vi "Diagnostics.Main.UUDT.Engine.vi"(8 "error in (no error)":errorcluster, 11 "State Variables":T1={"Comm"=refnum, "Parameters"={"Properties"={"Name"="", "CAN"={"CAN Interface"=enum."CAN1", "Baud Rate"=0, "Diagnostic Protocol"=enum."GMLAN", "Transport Protocol"=enum."ISO TP - Normal Mode", "Transmit ID"=0, "Receive ID"=0, "Transmit Extension"=2, "Receive Extension"=1, "Receive UUDT ID"=0, "Enable Stream"=TRUE, "VW TP Channel ID"=0, "Security"={"Source DLL Path"=path "", "Security Level"=0, "Target DLL Path"=path ""}, "Fill Frame"=FALSE, "Fill Byte"=255, "Termination"=FALSE}, "986x"={"Enable"=FALSE, "RIO Device"=0, "Bitfile"=path ""}, "Reads"=[], "Frames Lookup"=variant(enum16{"GMLAN", "KWP-2000", "UDS"} enum."GMLAN"), "Writes"=[], "DPIDs"=[], "DPID Lookup"=variant(u32 0), "DTC descriptor"={"DTC Byte Length"=2, "Status Byte Length"=1, "Add Data Byte Length"=1, "Byte Order"=enum."Motorola"}, "Created DTCs"=0}}, "ADCS Connection"={"Diag CAN Handle"=0, "Transport Protocol"=enum."ISO TP - Normal Mode", "Receive Address Extension"=0, "Transmit Address Extension"=0, "Receive CAN Id"=0, "Transmit CAN Id"=0, "Diag CAN Queue"=refnum, "Log Frames ?"=FALSE, "My TP Address"=0, "Other TP Address"=0, "T1"=0, "T2"=0, "T3"=0, "T4"=0, "Tx SN"=0, "Block Size"=0, "Rx SN"=0, "VW TP Initialized?"=FALSE, "Tx block no"=0, "baud rate"=0, "Interface"="", "Channel Diag CAN Handle"=0, "UDP Connection ID"=refnum, "TCP Connection ID"=refnum, "Target IP Addr"=0, "Source Address"=0, "Target Address"=0, "Send Header NACK?"=FALSE, "DLL Handle"=0, "NAD"=0, "Time Stamp read first"=0.0, "Time Stamp read last"=0.0, "Time Stamp write first"=0.0, "Time Stamp write last"=0.0, "Time Stamp write"=0.0, "Time Stamp read"=0.0}, "XNET References"={"Database"="", "GMLAN DPID Session"="", "Cluster"=""}, "XNETEngine (GMLAN)"=refnum, "Process"=refnum, "Reads"=refnum, "Writes"=refnum, "Cmds"=refnum, "DTCs"=refnum, "DTC Count"=refnum, "Status"=refnum, "Triggers"=refnum} {"Parameters"."Properties"."Writes"."Signals"."Byte Order" items=["Little Endian", "Big Endian"]; "Parameters"."Properties"."Writes"."Signals"."Data Type" items=["Signed", "Unsigned", "IEEE Float"]; "Parameters"."Properties"."CAN"."Fill Byte" format="%.0x"; "Parameters"."Properties"."CAN"."VW TP Channel ID" format="%.0x"; "Parameters"."Properties"."CAN"."Receive UUDT ID" format="%.0x"; "Parameters"."Properties"."CAN"."Receive Extension" format="%.0x"; "Parameters"."Properties"."CAN"."Transmit Extension" format="%.0x"; "Parameters"."Properties"."CAN"."Receive ID" format="%.0x"; "Parameters"."Properties"."CAN"."Transmit ID" format="%.0x"; "Parameters"."Properties"."Reads"."Signals"."Byte Order" items=["Little Endian", "Big Endian"]; "Parameters"."Properties"."Reads"."Signals"."Data Type" items=["Signed", "Unsigned", "IEEE Float"]}) -> (0 "error out":errorcluster)   [LabVIEW 2015, in "Diagnostics Addon Engine.lvlib"]
uses:
  Diagnostics Addon Engine.lvlib
  Types/Diagnostics.State.ctl
  <vilib>/NI/NIVS Inline Async API/_VS Inline Async API/Process/Process.lvclass
  <vilib>/NI/NIVS Addon Network Comm/Engine/VeriStand Comm.lvclass
  Shared/Types/SysDef.Compile.ctl
  Shared/Types/SysDef.Compile.Properties.ctl
  Shared/Types/CAN.ctl
  Shared/Types/CAN.Interface.ctl
  Shared/Types/Protocol.ctl
  Shared/Types/Transport.ctl
  Shared/Types/Security.ctl
  Shared/Types/986x.ctl
  Shared/Types/Frame.Compile.ctl
  Shared/Types/Type.ctl
  Shared/Types/Signal.ctl
  Shared/Types/DPID.ctl
  Shared/Types/DPID.Rate.ctl
  Shared/Types/DTCDescriptor.ctl
  <vilib>/Automotive Diagnostic Command Set/Diagnostic Transport.llb/Diag Reference.ctl
  <vilib>/Automotive Diagnostic Command Set/Diagnostic Transport.llb/Transport Protocol Selector.ctl
  <vilib>/Automotive Diagnostic Command Set/Diagnostic Transport.llb/Diag CAN Frame Log.ctl
  Types/XNET.Refs.ctl
  <vilib>/NI/AMC/Message Queue.ctl
  <vilib>/NI/AMC/Message.ctl
  <vilib>/NI/Tools/Keyed Array/KeyedArray.ctl
  <vilib>/NI/NIVS Inline Async API/_Data Access Engine/Data Access Engine/Types/Write.DVR.ctl
  <vilib>/NI/NIVS Inline Async API/_Data Access Engine/Access Type Classes/Write/Write.lvclass
  <vilib>/NI/NIVS Inline Async API/_Data Access Engine/Data Access Engine/Types/Read.DVR.ctl
  <vilib>/NI/NIVS Inline Async API/_Data Access Engine/Access Type Classes/Read/Read.lvclass
  <vilib>/NI/NIVS Inline Async API/_Data Access Engine/Data Access Engine/Types/ReadWrite.DVR.ctl
  <vilib>/NI/NIVS Inline Async API/_Data Access Engine/Access Type Classes/ReadWrite/ReadWrite.lvclass
  Types/DTC.ChangeCount.Info.ctl
  Shared/Types/DTC.Info.ctl
  <vilib>/xnet/xnet.llb/XNET Frame CAN.ctl
  <vilib>/xnet/xnet.llb/XNET Frame Type CAN.ctl
  <vilib>/NI/NIVS Inline Async API/_Data Access Engine/Access Type Classes/Write/Write.lvclass/Write.ctl
  Types/Frame.Data.ctl
  Shared/Types/DPID.Lookup.Info.ctl
  Shared/Types/DPID.Lookup.Info.PID.ctl
  Shared/Types/Frame.Lookup.Info.ctl
  <vilib>/NI/NIVS Addon Network Comm/Engine/VeriStand Comm.lvclass/VeriStand Comm.ctl
  <vilib>/NI/NIVS Inline Async API/_VS Inline Async API/Process/Process.lvclass/Process.ctl
  <vilib>/NI/NIVS Inline Async API/_Data Access Engine/Data Access Engine/Methods/Write.Data.vi
  <vilib>/NI/NIVS Inline Async API/_Data Access Engine/Data Access Engine/Methods/Write.Data.Commit.vi
  <vilib>/NI/NIVS Inline Async API/_Data Access Engine/Data Access Engine/Methods/Write.Data.Buffer.vi
  <vilib>/NI/NIVS Inline Async API/_Data Access Engine/Access Type Classes/Write/Write.ProcessData.vi
  <vilib>/NI/NIVS Inline Async API/_Data Access Engine/Access Type Classes/Write/Write.Commit.vi
  <vilib>/NI/NIVS Inline Async API/_Data Access Engine/Access Type Classes/Write/Write.Buffer.vi
  GMLAN/Utilities/Convert Raw Data to DTCs.vi
  <vilib>/NI/AMC/Send Local Message.vi
  <vilib>/NI/AMC/Read Termination Message.vi
  <vilib>/NI/NIVS Inline Async API/_VS Inline Async API/Error Handling Process/SubVIs/Error.ConvertArray.vi
  <vilib>/NI/AMC/Create Single Message.vi
  <vilib>/NI/AMC/Update Message Routing Info.vi
  <vilib>/NI/AMC/Send Message.vi
  <vilib>/Automotive Diagnostic Command Set/Diagnostic Protocols.llb/Convert to Phys.vi
  <vilib>/xnet/xnet.llb/XNET Convert (Frame Raw to Signal).vi
  <vilib>/xnet/xnet.llb/XNET Read (Frame CAN).vi
  <vilib>/xnet/xnet.llb/XNET Convert (Frame CAN to Signal).vi
  Shared/SubVIs/Constants.vi
  <vilib>/NI/AMC/Globals.vi
  Shared/Diagnostics Addon Shared.lvlib
  <vilib>/NI Veristand/Custom Device Tools/Custom Device Utility Library/Custom Device Utility Library.lvlib
  <vilib>/NI/AMC/AMC.lvlib
  GMLAN/GMLAN.lvlib
  <vilib>/NI/NIVS Inline Async API/_Data Access Engine/Data Access Engine/Data Access Engine.lvclass
  <vilib>/NI/Tools/Keyed Array/Tools_KeyedArray.lvlib
  <vilib>/addons/Automotive Diagnostic Command Set/NI_Automotive Diagnostic Command Set.lvlib
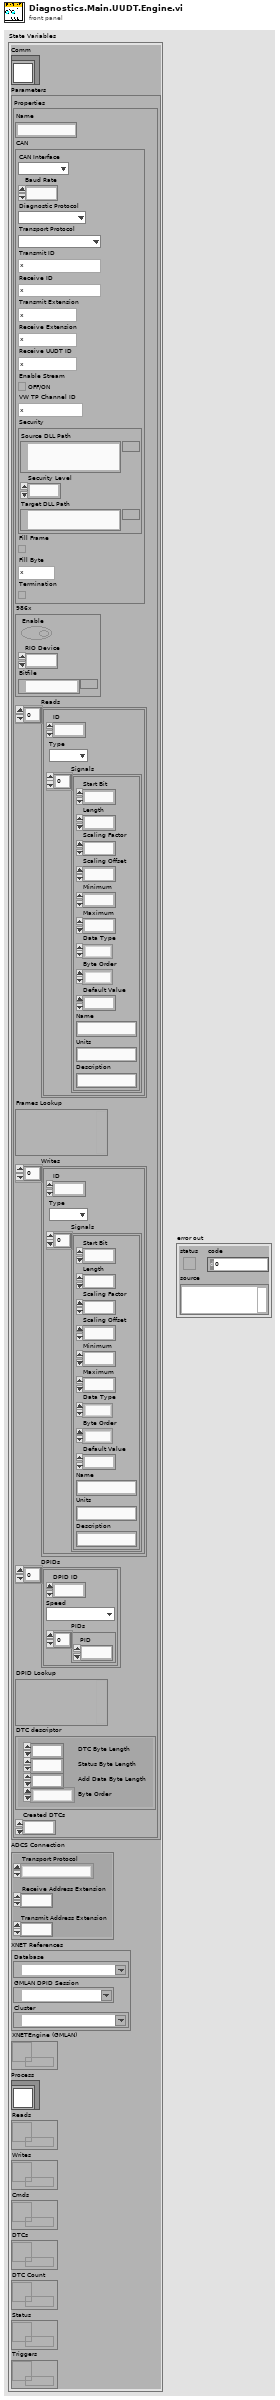
[diagram p1: front panel]
types:
  T1 = typedef "Diagnostics Addon Engine.lvlib/Diagnostics.State.ctl" = cluster{"Comm":refnum<class "VeriStand Comm.lvclass">, "Parameters":T2, "ADCS Connection":T16, "XNET References":T18, "XNETEngine (GMLAN)":T19, "Process":refnum<class "Process.lvclass">, "Reads":T20, "Writes":T21, "Cmds":T22, "DTCs":T20, "DTC Count":T20, "Status":T20, "Triggers":T22}
  T2 = typedef "Diagnostics Addon Shared.lvlib/SysDef.Compile.ctl" = cluster{"Properties":T3}
  T3 = typedef "Diagnostics Addon Shared.lvlib/SysDef.Compile.Properties.ctl" = cluster{"Name":string, "CAN":T4, "986x":T9, "Reads":T10[], "Frames Lookup":variant, "Writes":T10[], "DPIDs":T13[], "DPID Lookup":variant, "DTC descriptor":T15, "Created DTCs":u32}
  T4 = typedef "Diagnostics Addon Shared.lvlib/CAN.ctl" = cluster{"CAN Interface":T5, "Baud Rate":u32, "Diagnostic Protocol":T6, "Transport Protocol":T7, "Transmit ID":u32, "Receive ID":u32, "Transmit Extension":u8, "Receive Extension":u8, "Receive UUDT ID":u32, "Enable Stream":bool, "VW TP Channel ID":u32, "Security":T8, "Fill Frame":bool, "Fill Byte":u8, "Termination":bool}
  T5 = typedef "Diagnostics Addon Shared.lvlib/CAN.Interface.ctl" = enum16{"CAN0", "CAN1", "CAN2", "CAN3", "CAN4", "CAN5", "CAN6", "CAN7", "CAN8", "CAN9", "CAN10", "CAN11", "CAN12", "CAN13", "CAN14", "CAN15", "CAN16", "CAN17", "CAN18", "CAN19", "CAN20", "CAN21", "CAN22", "CAN23", "CAN24", "CAN25", "CAN26", "CAN27", "CAN28", "CAN29", "CAN30", "CAN31", "CAN32", "CAN33", "CAN34", "CAN35", "CAN36", "CAN37", "CAN38", "CAN39", "CAN40", "CAN41", "CAN42", "CAN43", "CAN44", "CAN45", "CAN46", "CAN47", "CAN48", "CAN49", "CAN50", "CAN51", "CAN52", "CAN53", "CAN54", "CAN55", "CAN56", "CAN57", "CAN58", "CAN59", "CAN60", "CAN61", "CAN62", "CAN63", "CAN 256 (Virtual)", "CAN 257 (Virtual)"}
  T6 = typedef "Diagnostics Addon Shared.lvlib/Protocol.ctl" = enum16{"GMLAN", "KWP-2000", "UDS", "User-Defined"}
  T7 = typedef "Diagnostics Addon Shared.lvlib/Transport.ctl" = enum16{"ISO TP - Normal Mode", "ISO TP - Mixed Mode", "VW TP 2.0", "Diagnostics on IP"}
  T8 = typedef "Diagnostics Addon Shared.lvlib/Security.ctl" = cluster{"Source DLL Path":path, "Security Level":u8, "Target DLL Path":path}
  T9 = typedef "Diagnostics Addon Shared.lvlib/986x.ctl" = cluster{"Enable":bool, "RIO Device":u16, "Bitfile":path}
  T10 = typedef "Diagnostics Addon Shared.lvlib/Frame.Compile.ctl" = cluster{"ID":u32, "Type":T11, "Signals":T12[]}
  T11 = typedef "Diagnostics Addon Shared.lvlib/Type.ctl" = enum16{"DID", "CDID", "PID", "CPID", "Read Memory", "Write Memory", "DTC Control", "IO Cmd", "IO Resp", "Routine Start Cmd", "Routine Start Resp", "Routine Request Cmd", "Routine Request Resp", "Routine Stop Cmd", "Routine Stop Resp", "UserDefined Cmd", "UserDefined Rsp"}
  T12 = typedef "Diagnostics Addon Shared.lvlib/Signal.ctl" = cluster{"Start Bit":u32, "Length":u32, "Scaling Factor":dbl, "Scaling Offset":dbl, "Minimum":dbl, "Maximum":dbl, "Data Type":u32, "Byte Order":u32, "Default Value":dbl, "Name":string, "Units":string, "Description":string}
  T13 = typedef "Diagnostics Addon Shared.lvlib/DPID.ctl" = cluster{"DPID ID":u8, "Speed":T14, "PIDs":u16[]}
  T14 = typedef "Diagnostics Addon Shared.lvlib/DPID.Rate.ctl" = enum16{"Slow", "Medium", "Fast"}
  T15 = typedef "Diagnostics Addon Shared.lvlib/DTCDescriptor.ctl" = cluster{"DTC Byte Length":i32, "Status Byte Length":i32, "Add Data Byte Length":i32, "Byte Order":enum16{"Motorola", "Intel"}}
  T16 = typedef "NI_Automotive Diagnostic Command Set.lvlib/Diag Reference.ctl" = cluster{"Diag CAN Handle":u32, "Transport Protocol":T17, "Receive Address Extension":u8, "Transmit Address Extension":u8, "Receive CAN Id":u32, "Transmit CAN Id":u32, "Diag CAN Queue":refnum<queue>, "Log Frames ?":bool, "My TP Address":u8, "Other TP Address":u8, "T1":u16, "T2":u16, "T3":u16, "T4":u16, "Tx SN":u8, "Block Size":u8, "Rx SN":u8, "VW TP Initialized?":bool, "Tx block no":u8, "baud rate":u32, "Interface":string, "Channel Diag CAN Handle":u32, "UDP Connection ID":refnum<k16>, "TCP Connection ID":refnum<k5>, "Target IP Addr":u32, "Source Address":u16, "Target Address":u16, "Send Header NACK?":bool, "DLL Handle":u32, "NAD":u8, "Time Stamp read first":dbl, "Time Stamp read last":dbl, "Time Stamp write first":dbl, "Time Stamp write last":dbl, "Time Stamp write":dbl, "Time Stamp read":dbl}
  T17 = typedef "NI_Automotive Diagnostic Command Set.lvlib/Transport Protocol Selector.ctl" = enum16{"ISO TP - Normal Mode", "ISO TP - Mixed Mode", "VW TP 2.0", "Diagnostics on IP", "ISO TP LIN"}
  T18 = typedef "Diagnostics Addon Engine.lvlib/XNET.Refs.ctl" = cluster{"Database":refnum<k21>, "GMLAN DPID Session":refnum<k21>, "Cluster":refnum<k21>}
  T19 = typedef "AMC.lvlib/Message Queue.ctl" = refnum<queue>
  T20 = typedef "Data Access Engine.lvlib/Data Access Engine.lvclass/Write.DVR.ctl" = refnum<data-value>
  T21 = typedef "Data Access Engine.lvlib/Data Access Engine.lvclass/Read.DVR.ctl" = refnum<data-value>
  T22 = typedef "Data Access Engine.lvlib/Data Access Engine.lvclass/ReadWrite.DVR.ctl" = refnum<data-value>
  T23 = typedef "Diagnostics Addon Shared.lvlib/DTC.Info.ctl" = cluster{"Timestamp":dbl, "DTC":dbl, "Status":dbl, "Add Data":dbl}
  T24 = typedef "Diagnostics Addon Engine.lvlib/DTC.ChangeCount.Info.ctl" = cluster{"DTCCountChange?":bool, "Timestamp":timestamp}
  T25 = typedef "XNET Frame CAN.ctl" = cluster{"timestamp":timestamp, "payload":u8[], "identifier":u32, "type":T26, "extended?":bool, "echo?":bool}
  T26 = typedef "XNET Frame Type CAN.ctl" = u8
  T27 = cluster{"Change DTC Count Cluster":T24, "Previous DTCs":T23[], "Prev DTC Frames":T25[]}
  T28 = typedef "Diagnostics Addon Engine.lvlib/Frame.Data.ctl" = cluster{"ID":u16, "Raw Frame":u8[]}
  T29 = typedef "Diagnostics Addon Shared.lvlib/DPID.Lookup.Info.ctl" = cluster{"PID Info":T30, "Datatable Lookup":T31, "Conversion":refnum<k21>}
  T30 = typedef "Diagnostics Addon Shared.lvlib/DPID.Lookup.Info.PID.ctl" = cluster{"PID":u16, "Frame Length":u8}
  T31 = typedef "Diagnostics Addon Shared.lvlib/Frame.Lookup.Info.ctl" = cluster{"Offset":i32, "Length":i32, "ByteLength":u16}
  T32 = typedef "Diagnostic Trouble Code.ctl" = cluster{"DTC":u32, "Status":u32, "Add Data":u32}
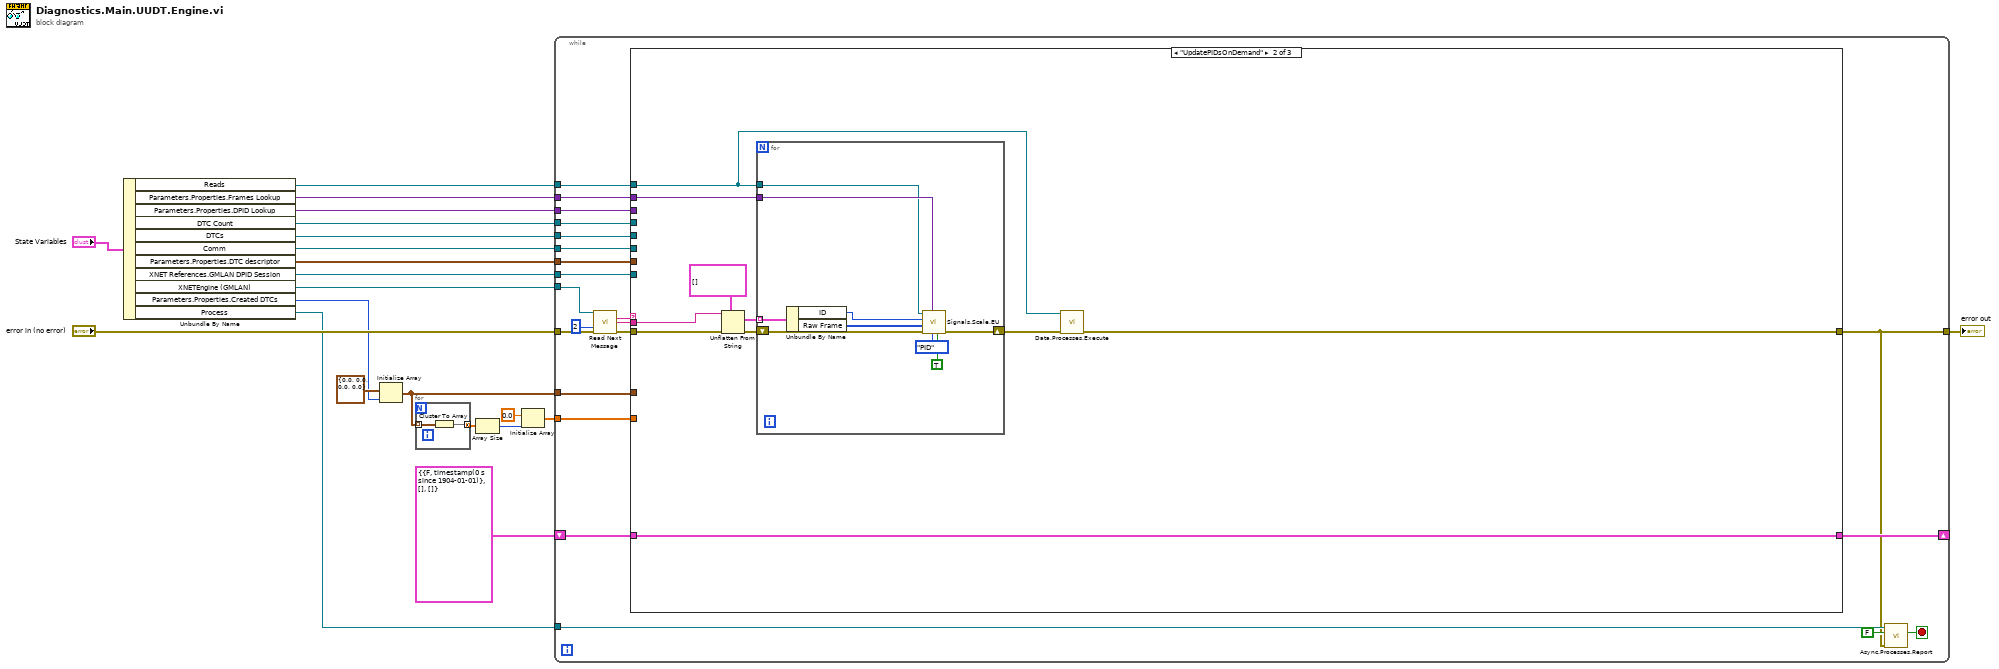
[diagram p0: block diagram]
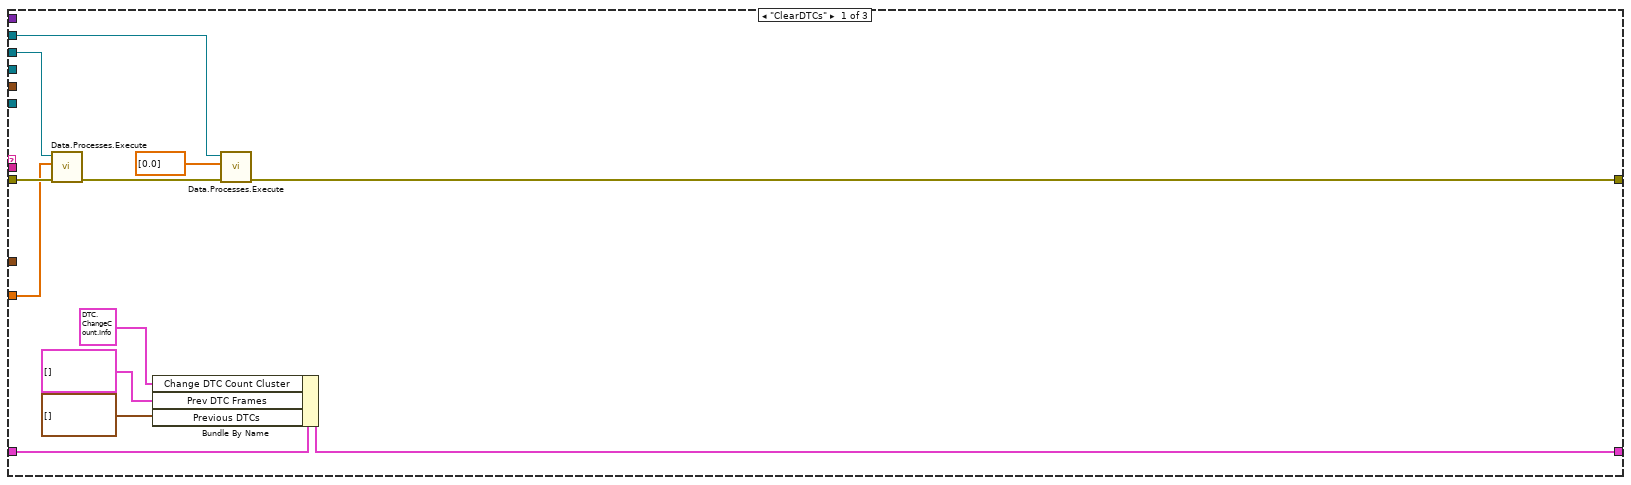
[diagram p2: hidden frame]
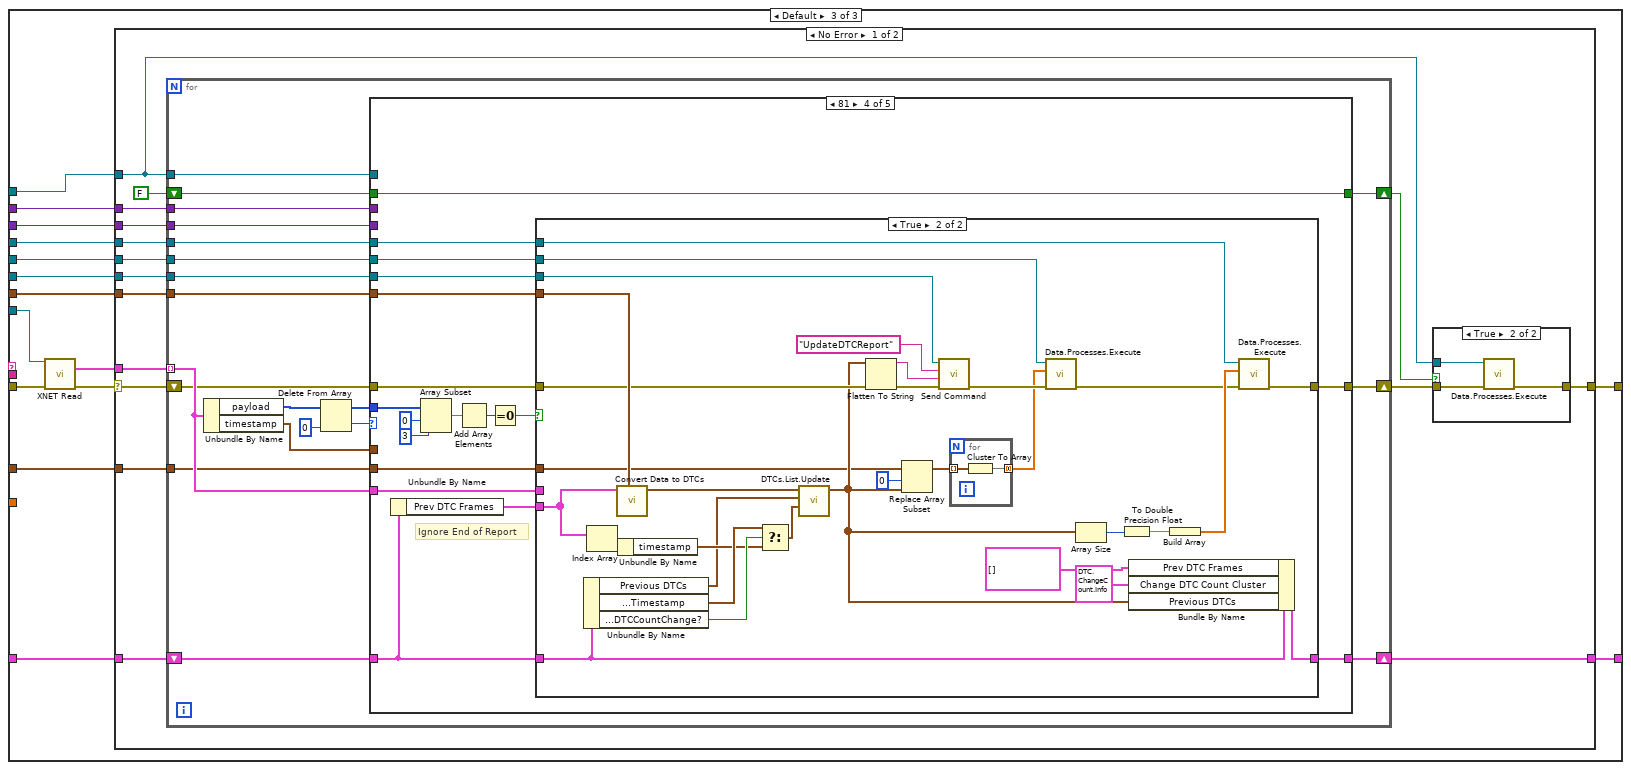
[diagram p3: hidden frame]
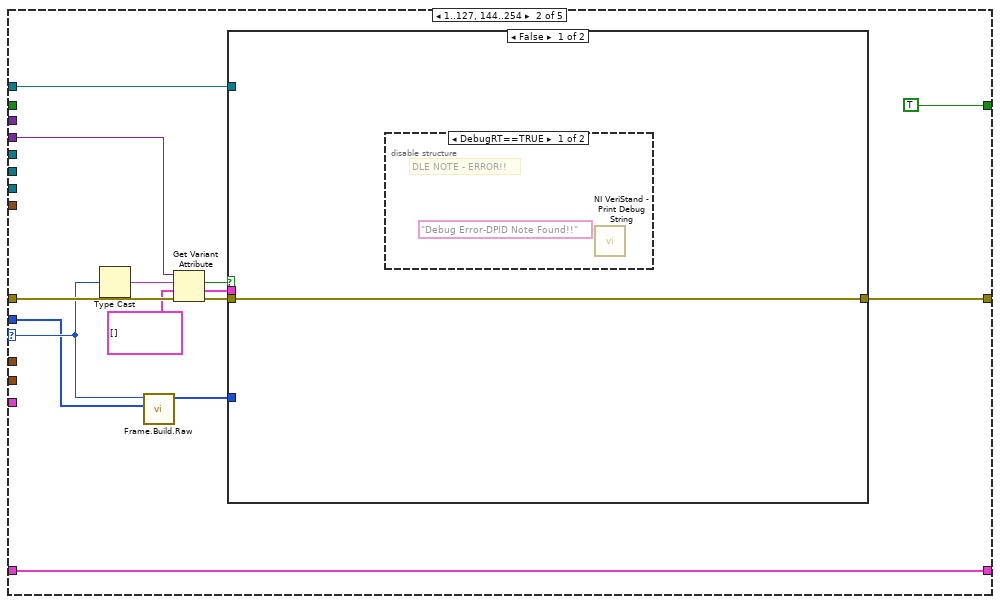
[diagram p5: hidden frame]
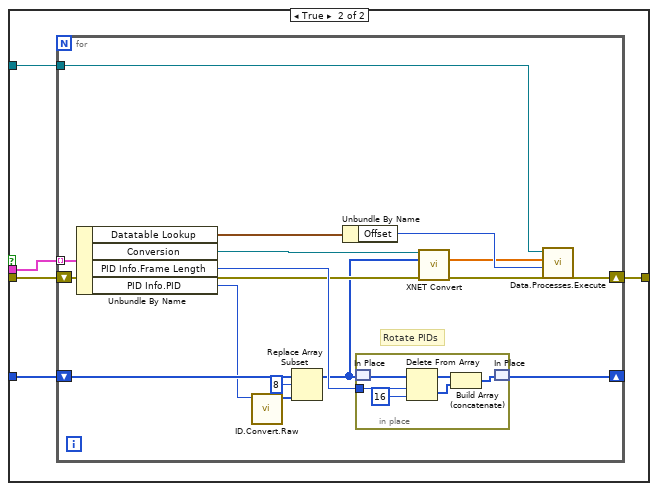
[diagram p7: hidden frame]
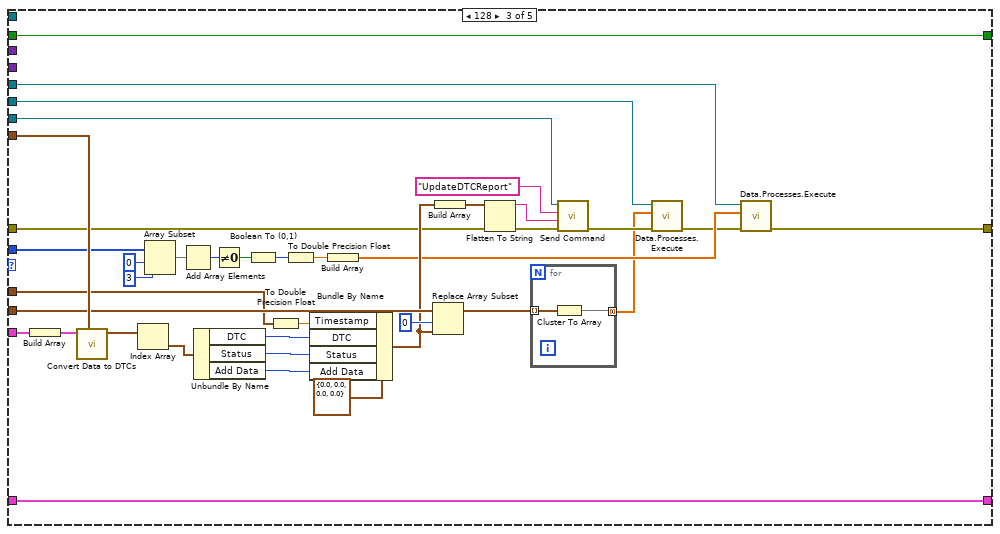
[diagram p8: hidden frame]
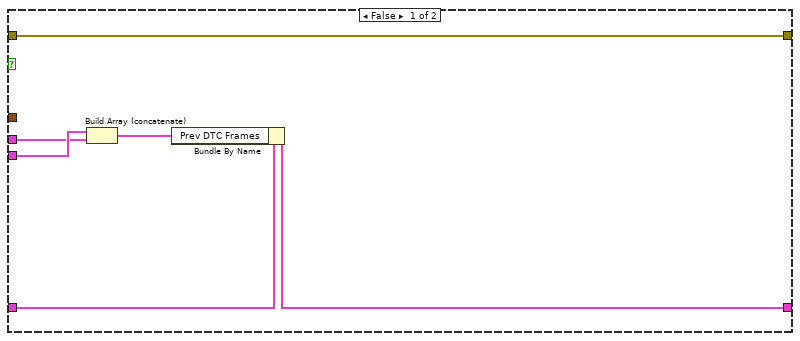
[diagram p9: hidden frame]
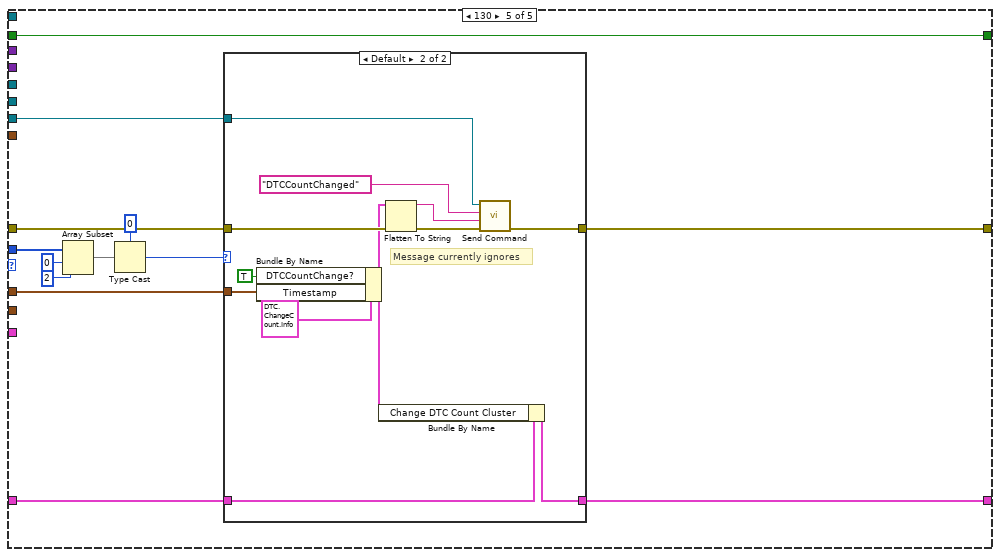
[diagram p10: hidden frame]
diagram:
  n1 = Unbundle By Name("State Variables") -> ("Reads"=w16:T20, "Parameters.Properties.Frames Lookup"=w15:variant, "Parameters.Properties.DPID Lookup"=w9:variant, "DTC Count"=w11:T20, "DTCs"=w19:T20, "Comm"=w18:refnum<class "VeriStand Comm.lvclass">, "Parameters.Properties.DTC descriptor"=w12:T15, "XNET References.GMLAN DPID Session"=w14:refnum<k21>, "XNETEngine (GMLAN)"=w8:T19, "Parameters.Properties.Created DTCs"=w7:u32, "Process"=w1:refnum<class "Process.lvclass">)
  n2 = Initialize Array(T23 {"Timestamp"=0.0, "DTC"=0.0, "Status"=0.0, "Add Data"=0.0} ("Diagnostic Trouble Code"), w7) -> (w6:T23[])
  n3 = for {
    tunnel: w6 -> [w23] mode=indexing
    tunnel: [w22] -> w3 mode=concatenating
    n4 = Cluster To Array(cluster=w23) -> (array=w22:dbl[])
  }
  n5 = Array Size(array=w3) -> (size(s)=w4:i32)
  n6 = Initialize Array(0.0 ("element"), w4) -> (w2:dbl[])
  n7 = while {
    tunnel: "error in (no error)" -> [w39]
    tunnel: [w26] -> w13
    tunnel: w12 -> [w45]
    tunnel: w14 -> [w44]
    tunnel: w15 -> [w43]
    tunnel: w16 -> [w42]
    tunnel: w18 -> [w41]
    tunnel: w1 -> [w28]
    tunnel: w8 -> [w33]
    shift-right: [w35] -> _
    shift-left: T27 {"Change DTC Count Cluster"={"DTCCountChange?"=FALSE, "Timestamp"=timestamp(0 s since 1904-01-01)}, "Previous DTCs"=[], "Prev DTC Frames"=[]} -> [w36]
    tunnel: w19 -> [w34]
    tunnel: w11 -> [w32]
    tunnel: w6 -> [w31]
    tunnel: w9 -> [w30]
    tunnel: w2 -> [w24]
    stop <- w25 stop-if-true
    n8 = call <vilib>:"Read Next Message.vi"("message queue in"=w33, "timeout (1 ms)"=2 ("timeout (1ms)"), "error in"=w39) -> ("message name"=w37:string, "message value"=w29:string, "error out"=w38:errorcluster)  [unwired: 5 in, 5 out]
    n9 = case shown="\"UpdatePIDsOnDemand\"" w37 {
      tunnel: [w48 w59 w89] -> w26
      tunnel: w45 -> [_ _ w88]
      tunnel: w38 -> [w47 w67 w87]
      tunnel: w44 -> [_ _ w86]
      tunnel: w43 -> [_ w62 w85]
      tunnel: w42 -> [_ w58 w84]
      tunnel: w41 -> [_ _ w83]
      tunnel: w36 -> [w57 w61 w82]
      tunnel: [w56 w61 w81] -> w35
      tunnel: w34 -> [w52 _ w80]
      tunnel: w32 -> [w50 _ w79]
      tunnel: w31 -> [_ _ w78]
      tunnel: w30 -> [_ _ w77]
      tunnel: w29 -> [_ w66 _]
      tunnel: w24 -> [w46 _ _]
      frame "ClearDTCs" {
        n10 = call-poly <vilib>:"Data.Processes.Execute.vi"("error in (no error)"=w47, "Values"=w46, "Ref"=w52) -> ("error out"=w49:errorcluster)  [unwired: 8 in]
        n11 = Bundle By Name(cluster=w57, "Change DTC Count Cluster"=T24 {"DTCCountChange?"=FALSE, "Timestamp"=timestamp(0 s since 1904-01-01)}, "Prev DTC Frames"=T25[] [] ("Previous DTC Frames"), "Previous DTCs"=T23[] []) -> (w56:T27)
        n12 = call-poly <vilib>:"Data.Processes.Execute.vi"("error in (no error)"=w49, "Values"=dbl[] [0.0] ("element"), "Ref"=w50) -> ("error out"=w48:errorcluster)  [unwired: 8 in]
      }
      frame "UpdatePIDsOnDemand" {
        n13 = Unflatten From String(type=T28[] [], binary string=w66, error in (no error)=w67) -> (value=w63:T28[], error out=w64:errorcluster)  [unwired: 2 in, 1 out]
        n14 = for {
          shift-right: [w72] -> w60
          shift-left: w64 -> [w73]
          tunnel: w63 -> [w76] mode=indexing
          tunnel: w62 -> [w71]
          tunnel: w58 -> [w69]
          n15 = Unbundle By Name(w76) -> ("ID"=w75:u16, "Raw Frame"=w74:u8[])
          n16 = call "Signals.Scale.EU.vi"("Buffer?"=TRUE, "Type"=Type."PID", "Lookup"=w71, "error in (no error)"=w73, "Unscaled Data"=w74, "ID"=w75, "Reads Ref"=w69) -> ("error out"=w72:errorcluster)  [unwired: 4 in]
        }
        n17 = call-poly <vilib>:"Data.Processes.Execute.vi"("error in (no error)"=w60, "Ref"=w58) -> ("error out"=w59:errorcluster)  [unwired: 9 in]
      }
      frame Default {
        n18 = call-poly <vilib>:"XNET Read.vi"("session in"=w86, "error in (no error)"=w87) -> ("data"=w90:T25[], "error out"=w91:errorcluster)  [unwired: 10 in, 2 out]
        n19 = case shown="No Error" w91 {
          selector: w91 -> [w106 w303]
          tunnel: w90 -> [w107 _]
          tunnel: [w102 w303] -> w89
          tunnel: w88 -> [w104 _]
          tunnel: w85 -> [w103 _]
          tunnel: w84 -> [w92 _]
          tunnel: w83 -> [w101 _]
          tunnel: w82 -> [w98 w302]
          tunnel: [w97 w302] -> w81
          tunnel: w80 -> [w96 _]
          tunnel: w79 -> [w95 _]
          tunnel: w78 -> [w94 _]
          tunnel: w77 -> [w93 _]
          frame No Error {
            n20 = for {
              tunnel: w107 -> [w127] mode=indexing
              shift-right: [w109] -> w105
              shift-left: w106 -> [w110]
              tunnel: w104 -> [w126]
              tunnel: w103 -> [w125]
              tunnel: w101 -> [w124]
              shift-right: [w121] -> w99
              shift-left: FALSE -> [w122]
              shift-right: [w120] -> w97
              shift-left: w98 -> [w119]
              tunnel: w96 -> [w118]
              tunnel: w95 -> [w117]
              tunnel: w94 -> [w116]
              tunnel: w93 -> [w115]
              tunnel: w92 -> [w108]
              n21 = Unbundle By Name(w127) -> ("payload"=w113:u8[], "timestamp"=w123:timestamp)
              n22 = Delete From Array(array=w113, index=0) -> (deleted portion=w111:u8, array with subset deleted=w112:u8[])  [unwired: 1 in]
              n23 = case shown="81" w111 {
                selector: w111 -> [_ w133 _ _ _]
                tunnel: w112 -> [_ w132 w202 w231 w281]
                tunnel: w127 -> [_ _ w211 w215 _]
                tunnel: [w130 w144 w176 w223 w278] -> w109
                tunnel: w110 -> [w130 w141 w181 w224 w277]
                tunnel: w126 -> [_ _ w209 w225 _]
                tunnel: w125 -> [_ _ _ _ _]
                tunnel: w124 -> [_ _ w184 w218 w271]
                tunnel: w123 -> [_ _ w189 _ w276]
                tunnel: w122 -> [w129 _ w208 w220 w275]
                tunnel: [w129 TRUE w208 w220 w275] -> w121
                tunnel: [w128 w142 w207 w222 w273] -> w120
                tunnel: w119 -> [w128 w142 w207 w221 w274]
                tunnel: w118 -> [_ _ w180 w219 _]
                tunnel: w117 -> [_ _ w178 w217 _]
                tunnel: w116 -> [_ _ w196 w214 _]
                tunnel: w115 -> [_ w135 _ _ _]
                tunnel: w108 -> [_ w131 _ _ _]
                frame Default {
                }
                frame 1..127, 144..254 {
                  n24 = Type Cast(x=w133) -> (*(type *) &x=w138:string)  [unwired: 1 in]
                  n25 = call "Frame.Build.Raw.vi"("Data"=w132, "identifier"=w133) -> ("Raw Frame"=w134:u8[])  [unwired: 9 in]
                  n26 = Get Variant Attribute(Variant=w135, name=w138, default value (empty Variant)=T29[] [], error in=w141) -> (found=w136:bool, value=w139:T29[], error out=w140:errorcluster)  [unwired: 1 out]
                  n27 = case shown="False" w136 {
                    tunnel: [w145 w151] -> w144
                    tunnel: w140 -> [w145 w150]
                    tunnel: w139 -> [_ w149]
                    tunnel: w134 -> [_ w148]
                    tunnel: w131 -> [_ w147]
                    frame False {
                      n28 = disable-structure shown="DebugRT==TRUE" {
                        frame condition #0 {
                          # "DLE NOTE - ERROR!!"
                          n29 = call <vilib>:"NI VeriStand - Print Debug String.vi"("Message"="Debug Error-DPID Note Found!!" ("Debug String")) -> ()  [unwired: 10 in, 1 out]
                        }
                        frame condition #1 (active) {
                        }
                      }
                    }
                    frame True {
                      n30 = for {
                        shift-right: [w152] -> w151
                        shift-left: w150 -> [w162]
                        tunnel: w149 -> [w167] mode=indexing
                        shift-right: [w164] -> _
                        shift-left: w148 -> [w165]
                        tunnel: w147 -> [w156]
                        # "Rotate PIDs"
                        n31 = Unbundle By Name(w167) -> ("Datatable Lookup"=w161:T31, "Conversion"=w163:refnum<k21>, "PID Info.Frame Length"=w166:u8, "PID Info.PID"=w160:u16)
                        n32 = call "ID.Convert.Raw.vi"("identifier"=w160) -> ("Data"=w158:u8[])  [unwired: 10 in]
                        n33 = Replace Array Subset(array=w165, new element=w158, index=8) -> (w159:u8[])
                        n34 = Unbundle By Name(w161) -> ("Offset"=w155:i32)
                        n35 = in-place {
                          in-place-border: w166 -> [w172]
                          n36 = in-place-match #1(w159) -> (w171:u8[])
                          n37 = Delete From Array(array=w171, length=w172, index=16 ("length")) -> (deleted portion=w169:u8[], array with subset deleted=w170:u8[])
                          n38 = Build Array (concatenate)(w170, w169) -> (w168:u8[])
                          n39 = in-place-match #1(w168) -> (w164:u8[])
                        }
                        n40 = call-poly <vilib>:"XNET Convert.vi"("session in"=w163, "frame data"=w159, "error in (no error)"=w162) -> ("signal data"=w154:dbl[], "error out"=w153:errorcluster)  [unwired: 10 in, 1 out]
                        n41 = call-poly <vilib>:"Data.Processes.Execute.vi"("error in (no error)"=w153, "Offset"=w155, "Values"=w154, "Ref"=w156) -> ("error out"=w152:errorcluster)  [unwired: 7 in]
                      }
                    }
                  }
                }
                frame 128 {
                  n42 = Build Array(w211) -> (w210:T25[])
                  n43 = call "Convert Data to DTCs.vi"("DTC descriptor"=w209, "All DTCs"=w210) -> ("DTCs"=w195:T32[])  [unwired: 8 in, 1 out]
                  n44 = Index Array(array=w195) -> (element=w193:T32)  [unwired: 1 in]
                  n45 = Array Subset(array=w202, index=0, length=3) -> (w204:u8[])
                  n46 = Add Array Elements(numeric array=w204) -> (sum=w203:u8)
                  n47 = Unbundle By Name(w193) -> ("DTC"=w190:u32, "Status"=w191:u32, "Add Data"=w192:u32)
                  n48 = Not Equal To 0?(x=w203) -> (x != 0?=w201:bool)
                  n49 = Boolean To (0,1)(Boolean=w201) -> (0, 1=w200:i16)
                  n50 = To Double Precision Float(number=w189) -> (double precision float=w188:dbl)
                  n51 = To Double Precision Float(number=w200) -> (double precision float=w199:dbl)
                  n52 = Bundle By Name(cluster=T23 {"Timestamp"=0.0, "DTC"=0.0, "Status"=0.0, "Add Data"=0.0} ("Diagnostic Trouble Code"), "Timestamp"=w188, "DTC"=w190, "Status"=w191, "Add Data"=w192) -> (w183:T23)
                  n53 = Build Array(w199) -> (w179:dbl[])
                  n54 = Replace Array Subset(array=w196, new element=w183, index=0) -> (w197:T23[])
                  n55 = Build Array(w183) -> (w182:T23[])
                  n56 = Flatten To String(anything=w182, error in (no error)=w181) -> (data string=w185:string, error out=w186:errorcluster)  [unwired: 2 in, 1 out]
                  n57 = for {
                    tunnel: w197 -> [w213] mode=indexing
                    tunnel: [w212] -> w174 mode=concatenating
                    n58 = Cluster To Array(cluster=w213) -> (array=w212:dbl[])
                  }
                  n59 = call <vilib>:"Send Command.vi"("error in (no error)"=w186, "message value"=w185, "message name"="UpdateDTCReport" ("Message Name"), "VeriStand Comm in"=w184) -> ("error out"=w175:errorcluster)  [unwired: 6 in, 1 out]
                  n60 = call-poly <vilib>:"Data.Processes.Execute.vi"("error in (no error)"=w175, "Values"=w174, "Ref"=w180) -> ("error out"=w177:errorcluster)  [unwired: 8 in]
                  n61 = call-poly <vilib>:"Data.Processes.Execute.vi"("error in (no error)"=w177, "Values"=w179, "Ref"=w178) -> ("error out"=w176:errorcluster)  [unwired: 8 in]
                }
                frame 129 {
                  # "Ignore End of Report"
                  n62 = Unbundle By Name(w221) -> ("Prev DTC Frames"=w216:T25[])
                  n63 = Array Subset(array=w231, index=0, length=3) -> (w228:u8[])
                  n64 = Add Array Elements(numeric array=w228) -> (sum=w227:u8)
                  n65 = Equal To 0?(x=w227) -> (x = 0?=w226:bool)
                  n66 = case shown="True" w226 {
                    tunnel: w225 -> [_ w268]
                    tunnel: w218 -> [_ w245]
                    tunnel: w224 -> [w237 w261]
                    tunnel: [w237 w240] -> w223
                    tunnel: w221 -> [w236 w260]
                    tunnel: [w235 w258] -> w222
                    tunnel: w219 -> [_ w243]
                    tunnel: w217 -> [_ w241]
                    tunnel: w216 -> [w234 w248]
                    tunnel: w215 -> [w233 _]
                    tunnel: w214 -> [_ w246]
                    frame False {
                      n67 = Build Array (concatenate)(w234, w233) -> (w232:T25[])
                      n68 = Bundle By Name(cluster=w236, "Prev DTC Frames"=w232) -> (w235:T27)
                    }
                    frame True {
                      n69 = Unbundle By Name(w260) -> ("Previous DTCs"=w251:T23[], "Change DTC Count Cluster.Timestamp"=w256:timestamp, "Change DTC Count Cluster.DTCCountChange?"=w267:bool)
                      n70 = Index Array(array=w248) -> (element=w253:T25)  [unwired: 1 in]
                      n71 = call "Convert Data to DTCs.vi"("DTC descriptor"=w268, "All DTCs"=w248) -> ("DTCs"=w263:T32[])  [unwired: 8 in, 1 out]
                      n72 = Unbundle By Name(w253) -> ("timestamp"=w252:timestamp)
                      n73 = Select(t=w256, s=w267, f=w252) -> (s? t:f=w262:timestamp)
                      n74 = call "DTCs.List.Update.vi"("current time"=w262, "Previous Changed DTCs"=w251, "current DTCs"=w263) -> ("Active DTCs"=w247:T23[])  [unwired: 8 in]
                      n75 = Flatten To String(anything=w247, error in (no error)=w261) -> (data string=w264:string, error out=w265:errorcluster)  [unwired: 2 in, 1 out]
                      n76 = Replace Array Subset(array=w246, new element=w247, index=0) -> (w254:T23[])
                      n77 = call <vilib>:"Send Command.vi"("error in (no error)"=w265, "message value"=w264, "message name"="UpdateDTCReport" ("Message Name"), "VeriStand Comm in"=w245) -> ("error out"=w239:errorcluster)  [unwired: 6 in, 1 out]
                      n78 = for {
                        tunnel: w254 -> [w270] mode=indexing
                        tunnel: [w269] -> w238 mode=concatenating
                        n79 = Cluster To Array(cluster=w270) -> (array=w269:dbl[])
                      }
                      n80 = call-poly <vilib>:"Data.Processes.Execute.vi"("error in (no error)"=w239, "Values"=w238, "Ref"=w243) -> ("error out"=w242:errorcluster)  [unwired: 8 in]
                      n81 = Array Size(array=w247) -> (size(s)=w250:i32)
                      n82 = To Double Precision Float(number=w250) -> (double precision float=w249:dbl)
                      n83 = Bundle By Name(cluster=w260, "Prev DTC Frames"=T25[] [] ("data"), "Change DTC Count Cluster"=T24 {"DTCCountChange?"=FALSE, "Timestamp"=timestamp(0 s since 1904-01-01)}, "Previous DTCs"=w247) -> (w258:T27)
                      n84 = Build Array(w249) -> (w244:dbl[])
                      n85 = call-poly <vilib>:"Data.Processes.Execute.vi"("error in (no error)"=w242, "Values"=w244, "Ref"=w241) -> ("error out"=w240:errorcluster)  [unwired: 8 in]
                    }
                  }
                }
                frame 130 {
                  n86 = Array Subset(array=w281, index=0, length=2) -> (w280:u8[])
                  n87 = Type Cast(type=u16 0 ("length"), x=w280) -> (*(type *) &x=w272:u16)
                  n88 = case shown="Default" w272 {
                    tunnel: [w285 w297] -> w278
                    tunnel: w277 -> [w285 w294]
                    tunnel: w276 -> [_ w293]
                    tunnel: w274 -> [w284 w289]
                    tunnel: [w284 w288] -> w273
                    tunnel: w271 -> [_ w286]
                    frame 0 {
                      # "ChangeDTCCount Disabled."
                    }
                    frame Default {
                      # "Message currently ignores"
                      n89 = Bundle By Name(cluster=T24 {"DTCCountChange?"=FALSE, "Timestamp"=timestamp(0 s since 1904-01-01)} ("Cluster"), "DTCCountChange?"=TRUE, "Timestamp"=w293) -> (w290:T24)
                      n90 = Bundle By Name(cluster=w289, "Change DTC Count Cluster"=w290) -> (w288:T27)
                      n91 = Flatten To String(anything=w290, error in (no error)=w294) -> (data string=w296:string, error out=w295:errorcluster)  [unwired: 2 in, 1 out]
                      n92 = call <vilib>:"Send Command.vi"("error in (no error)"=w295, "message value"=w296, "message name"="DTCCountChanged" ("Message Name"), "VeriStand Comm in"=w286) -> ("error out"=w297:errorcluster)  [unwired: 6 in, 1 out]
                    }
                  }
                }
              }
            }
            n93 = case shown="True" w99 {
              tunnel: w105 -> [w298 w300]
              tunnel: [w298 w301] -> w102
              tunnel: w92 -> [_ w299]
              frame False {
              }
              frame True {
                n94 = call-poly <vilib>:"Data.Processes.Execute.vi"("error in (no error)"=w300, "Ref"=w299) -> ("error out"=w301:errorcluster)  [unwired: 9 in]
              }
            }
          }
          frame Error {
          }
        }
      }
    }
    n95 = call <vilib>:"Async.Processes.Report.vi"("Error"=w26, "Stop Async on Error?"=FALSE ("Stop on Error?"), "Process in"=w28) -> ("Stop"=w25:bool)  [unwired: 7 in, 1 out]
  }
  "error out" <- w13
